vi "RGB WS2812 Control VI.vi"() -> ()   [LabVIEW 2014]
uses:
  VI States.ctl
  <vilib>/Instr/_visa.llb/VISA Configure Serial Port (Instr).vi
panel:
  in  "Stop Button":bool
  in  "VISA resource name":refnum<visa-resource-name>
  in  "Color Box":u32(colorbox)
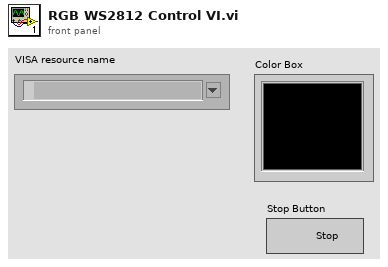
[diagram p1: front panel]
types:
  T1 = typedef "VI States.ctl" = enum16{"Poll", "Init Serial", "Read Serial", "Write Serial", "Close Serial"}
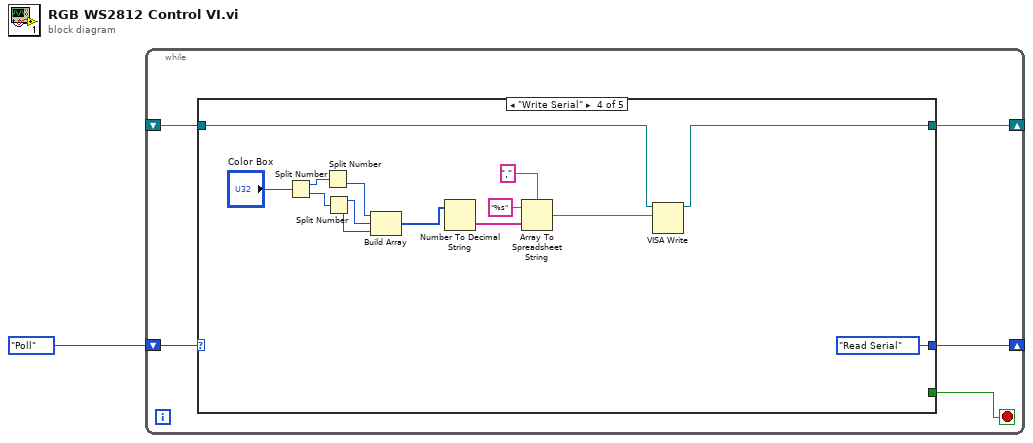
[diagram p0: block diagram]
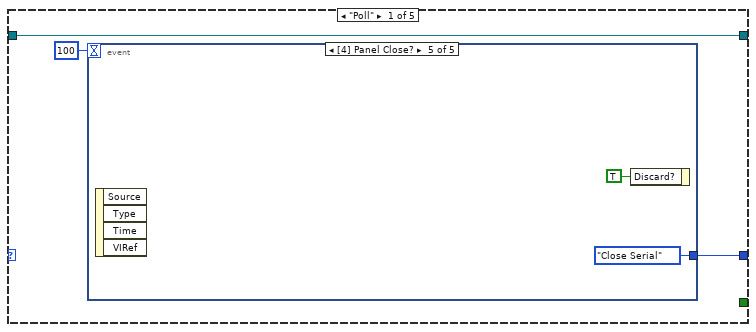
[diagram p2: hidden frame]
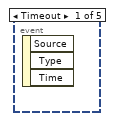
[diagram p3: hidden frame]
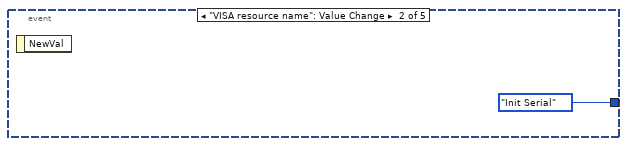
[diagram p4: hidden frame]
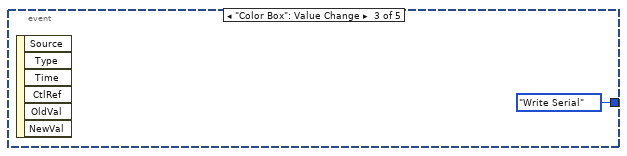
[diagram p5: hidden frame]
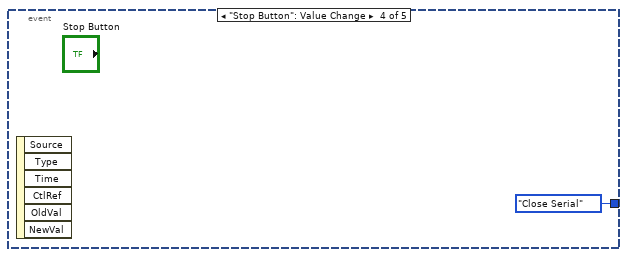
[diagram p6: hidden frame]
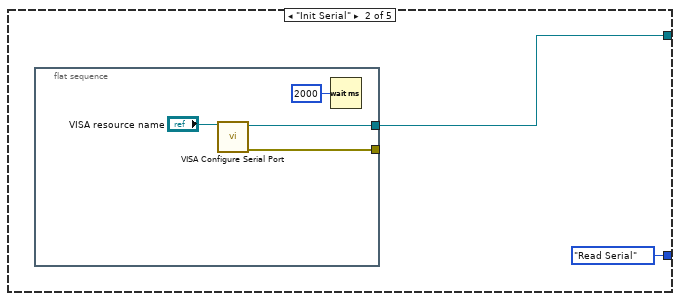
[diagram p7: hidden frame]
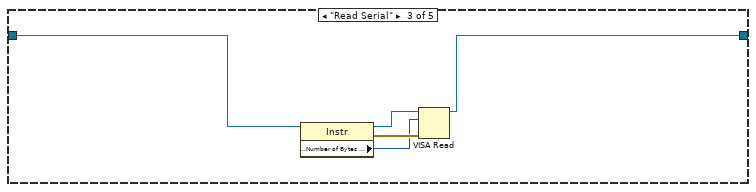
[diagram p8: hidden frame]
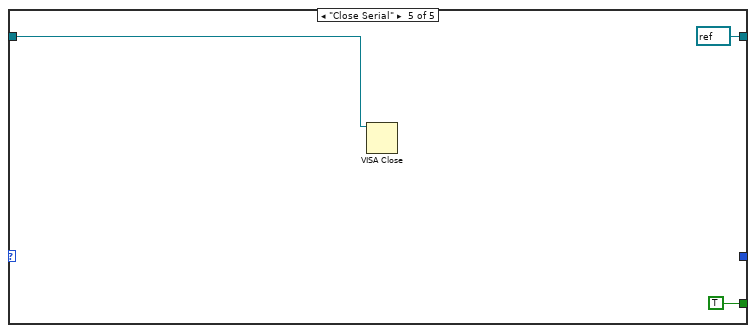
[diagram p9: hidden frame]
diagram:
  n1 = while {
    shift-right: [w5] -> _
    shift-left: VI_States."Poll" -> [w6]
    shift-right: [w4] -> _
    shift-left: _ -> [w3]
    stop <- w2 stop-if-true
    n2 = case shown="\"Write Serial\"" w6 {
      tunnel: [w8 VI_States."Read Serial" _ VI_States."Read Serial" _] -> w5
      tunnel: [w7 w16 w21 w38 refnum<visa-resource-name> refnum ("VISA resource name out")] -> w4
      tunnel: w3 -> [w7 _ w22 w39 w42]
      tunnel: [_ _ _ _ TRUE] -> w2
      frame "Poll" {
        n3 = event shown="[4] Panel Close?" {
          selector: _ -> [_ _ _ _ _]
          dyn-events: _ -> [_ _ _ _ _]
          timeout: 100 -> [_ _ _ _ _]
          tunnel: [_ VI_States."Init Serial" VI_States."Write Serial" VI_States."Close Serial" VI_States."Close Serial"] -> w8
          event Timeout {
            n4 = event-data() -> ()  [unwired: 1 in, 3 out]
          }
          event "VISA resource name": Value Change {
            n5 = event-data() -> ()  [unwired: 1 in, 1 out]
          }
          event "Color Box": Value Change {
            n6 = event-data() -> ()  [unwired: 1 in, 6 out]
          }
          event "Stop Button": Value Change {
            n7 = event-data() -> ()  [unwired: 1 in, 6 out]
          }
          event Panel Close? {
            n8 = event-data() -> ()  [unwired: 1 in, 4 out]
            n9 = event-data("Discard?"=TRUE) -> ()  [unwired: 1 in, 1 out]
          }
        }
      }
      frame "Init Serial" {
        n10 = flat-sequence {
          tunnel: [w20] -> w16
          tunnel: [w19] -> _
          frame #0 {
            n11 = call-poly "VISA Configure Serial Port"("VISA resource name"="VISA resource name") -> ("VISA resource name out"=w20:refnum<visa-resource-name>, "error out"=w19:errorcluster)  [unwired: 8 in, 5 out]
            n12 = Wait (ms)(milliseconds to wait=u32 2000) -> ()  [unwired: 1 out]
          }
        }
      }
      frame "Read Serial" {
        n13 = property class="Instr"(reference=w22) -> (reference out=w25:refnum<visa-resource-name>, error out=w24:errorcluster, "Serial Settings:Number of Bytes at Serial Port"=w23:u32)  [unwired: 1 in]
        n14 = VISA Read(VISA resource name=w25, byte count=w23, error in (no error)=w24) -> (VISA resource name out=w21:refnum<visa-resource-name>)  [unwired: 3 out]
      }
      frame "Write Serial" {
        n15 = Split Number(x="Color Box") -> (hi(x)=w36:u16, lo(x)=w35:u16)
        n16 = Split Number(x=w36) -> (lo(x)=w34:u8)  [unwired: 1 out]
        n17 = Split Number(x=w35) -> (hi(x)=w33:u8, lo(x)=w32:u8)
        n18 = Build Array(w34, w33, w32) -> (w26:u8[])
        n19 = Number To Decimal String(number=w26) -> (decimal integer string=w27:string[])  [unwired: 1 in]
        n20 = Array To Spreadsheet String(delimiter (Tab)=",", array=w27, 3:"%s" ("format string")) -> (spreadsheet string=w29:string)
        n21 = VISA Write(VISA resource name=w39, write buffer=w29) -> (VISA resource name out=w38:refnum<visa-resource-name>)  [unwired: 1 in, 2 out]
      }
      frame "Close Serial" {
        n22 = VISA Close(VISA resource name=w42) -> ()  [unwired: 1 in, 1 out]
      }
    }
  }
